vi "Day 3 Task 1.vi"() -> ()   [LabVIEW 2018]
panel:
  out "power consumption":u32
  out "epsilon number":u32
  out "gamma number":u32
  out "gamma rate":i32[](array[numeric])
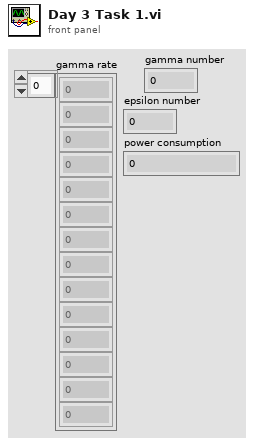
[diagram p1: front panel]
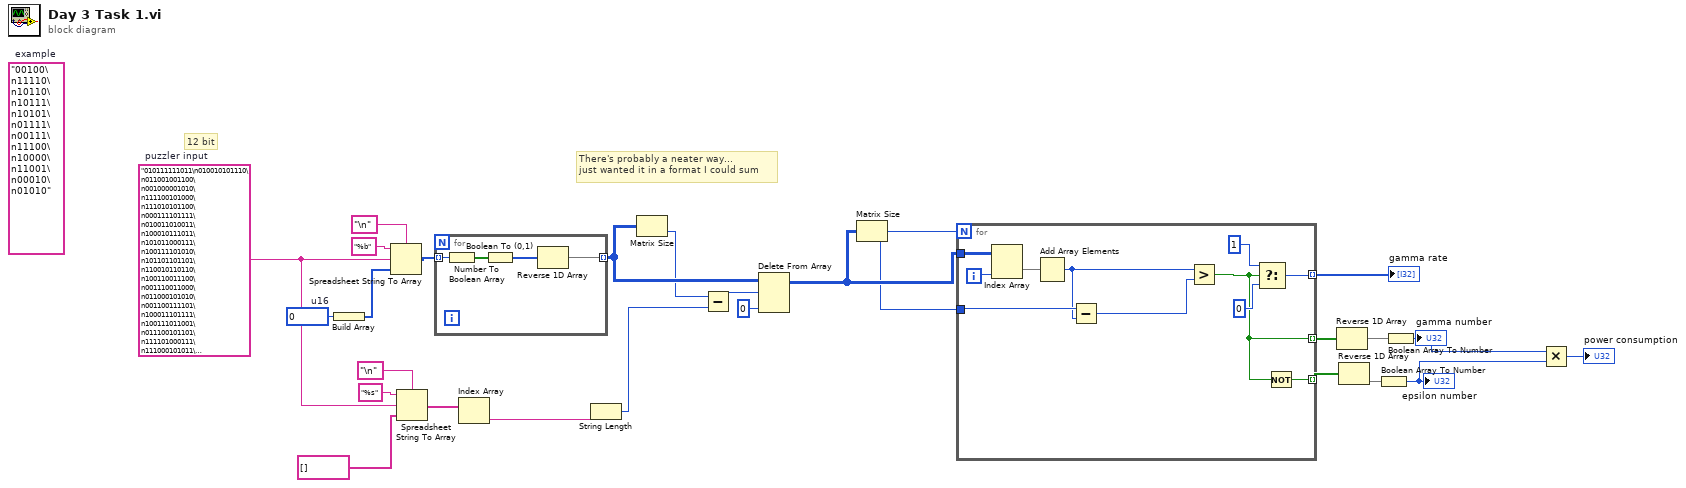
[diagram p0: block diagram]
diagram:
  w1 = "010111111011\n010010101110\n011001001100\n001000001010\n111100101000\n111010101100\n000111101111\n010011010011\n100010111011\n101011000111\n100111101010\n101101101101\n110010110110\n100110011100\n001110011000\n011000101010\n001100111101\n100011101111\n100111011001\n011100101101\n111101000111\n111000101011\n001001000101\n010110011000\n110100100001\n010010010011\n100100100100\n011011001000\n111101011101\n101011110011\n110011101101\n001001000100\n100111101110\n101101101010\n111110101000\n111011011001\n111110101101\n110101010100\n011100110000\n000010111110\n111011111111\n010111111110\n101001110101\n001111010100\n001111110001\n000010000000\n01..."  # puzzler input
  w25 = u16 0  # u16
  (unwired) "00100\n11110\n10110\n10111\n10101\n01111\n00111\n11100\n10000\n11001\n00010\n01010"  # example
  # "12 bit"
  # "There's probably a neater way...\njust wanted it in a format I could sum"
  n1 = Build Array(w25) -> (w21:u16[])
  n2 = Spreadsheet String To Array(delimiter (Tab)="\n", format string="%b", spreadsheet string=w1, array type (2D Dbl)=w21) -> (array=w24:u16[])
  n3 = Spreadsheet String To Array(delimiter (Tab)="\n", format string="%s", spreadsheet string=w1, array type (2D Dbl)=string[] []) -> (array=w6:string[])
  n4 = for {
    tunnel: w24 -> [w31] mode=indexing
    tunnel: [w29] -> w23 mode=indexing
    n5 = Number To Boolean Array(number=w31) -> (Boolean array=w30:bool[])
    n6 = Boolean To (0,1)(Boolean=w30) -> (0, 1=w28:i16[])
    n7 = Reverse 1D Array(array=w28) -> (reversed array=w29:i16[])
  }
  n8 = Index Array(array=w6) -> (element=w5:string)  [unwired: 1 in]
  n9 = String Length(string=w5) -> (length=w3:i32)
  n10 = Matrix Size(0:w23) -> (2:w22:i32)  [unwired: 1 out]
  n11 = Subtract(x=w22, y=w3) -> (x-y=w4:i32)
  n12 = Delete From Array(array=w23, length=w4, index (col)=0 ("disabled index (col)")) -> (array with subset deleted=w18:i16[][])  [unwired: 1 in, 1 out]
  n13 = Matrix Size(0:w18) -> (1:w17:i32, 2:w19:i32)
  n14 = for {
    N: w19 -> [_]
    tunnel: w18 -> [w42]
    tunnel: w17 -> [w39]
    tunnel: [w36] -> w20 mode=indexing
    tunnel: [w33] -> w15 mode=indexing
    tunnel: [w32] -> w14 mode=indexing
    i -> [w41]
    n15 = Index Array(array=w42, index (col)=w41) -> (element=w40:i16[])  [unwired: 1 in]
    n16 = Add Array Elements(numeric array=w40) -> (sum=w38:i16)
    n17 = Subtract(x=w39, y=w38) -> (x-y=w37:i32)
    n18 = Greater?(x=w38, y=w37) -> (0:w33:bool)
    n19 = Select(t=1, s=w33, f=0 ("x-y")) -> (s? t:f=w36:i32)
    n20 = Not(x=w33) -> (.not. x?=w32:bool)
  }
  "gamma rate" <- w20
  n21 = Reverse 1D Array(array=w15) -> (reversed array=w16:bool[])
  n22 = Reverse 1D Array(array=w14) -> (reversed array=w13:bool[])
  n23 = Boolean Array To Number(Boolean array=w13) -> (number=w11:u32)
  "epsilon number" <- w11
  n24 = Boolean Array To Number(Boolean array=w16) -> (number=w12:u32)
  "gamma number" <- w12
  n25 = Multiply(x=w12, y=w11) -> (x*y=→"power consumption":u32)
